vi "01 Reading a voltage.vi"() -> ()   [LabVIEW 2019]
uses:
  <vilib>/Instr/_visa.llb/VISA Configure Serial Port (Instr).vi
panel:
  out "Connected":bool
  in  "stop":bool
  in  "Arduino code":string="/*\n  Analog input, analog output, serial output\n\n  Reads an analog input pin, maps the result to a range from 0 to 255 and uses\n  the result to set the pulse width modulation (PWM) of an output pin.\n  Also prints the results to the Serial Monitor.\n\n  The circuit:\n  - potentiometer connected to analog pin 0.\n    Center pin of the potentiometer goes to the analog pin.\n    side pins of the potentiometer go to +5V and ground\n  - LED connected from digital pin 9 to ground\n\n  created 29 Dec. 2008\n  modified 9 Apr 2012\n  by Tom Igoe\n\n  This example code is in the public domain.\n\n  http://www.arduino.cc/en/Tutorial/AnalogInOutSerial\n*/\n\n// These constants won't change. They're used to give names to the pins used:\nconst int analogInPin = A0;  // Analog input pin that the potentiometer is attached to\nconst int analogOutPin = 9; // Analog output pin that the LED is attached to\n\nint sensorValue = 0;        // value read from the pot\nint outputValue = 0;        // value output to the PWM (analog out)\n\nvoid setup() {\n  // initialize serial communications at 9600 bps:\n  Serial.begin(9600);\n}\n\nvoid loop() {\n  // read the analog in value:\n  sensorValue = analogRead(analogInPin);\n  // map it to the range of the analog out:\n  outputValue = map(sensorValue, 0, 1023, 0, 255);\n  // change the analog out value:\n  analogWrite(analogOutPin, outputValue);\n\n  // print the results to the Serial Monitor:\n  Serial.print(\"sensor = \");\n  Serial.print(sensorValue);\n  Serial.print(\"\\t output = \");\n  Serial.println(outputValue);\n\n  // wait 2 milliseconds before the next loop for the analog-to-digital\n  // converter to settle after the last reading:\n  delay(2);\n}"
  in  "Arduino Port":refnum<visa-resource-name>
  out "Gauge":i32(knob) scale=0.0..1000.0
  # "Download and run the Arduino Example Code AnalogInOutSerial (below)\nHit the Run arrow and see the Gauge change to the value of the sensor (read over serial)"
  # "Hit Cmd E to see the diagram (code)"
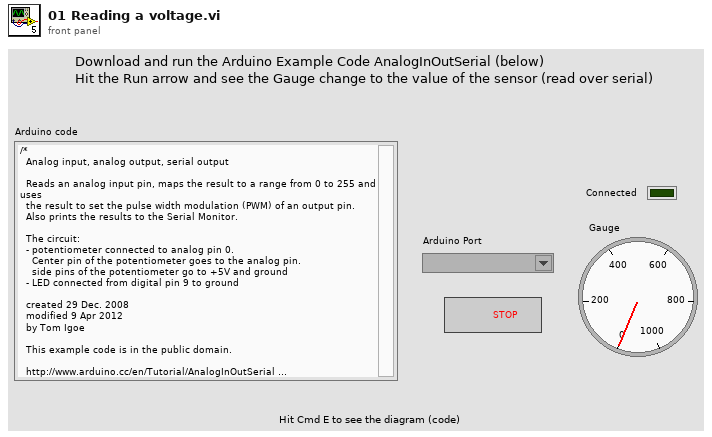
[diagram p1: front panel]
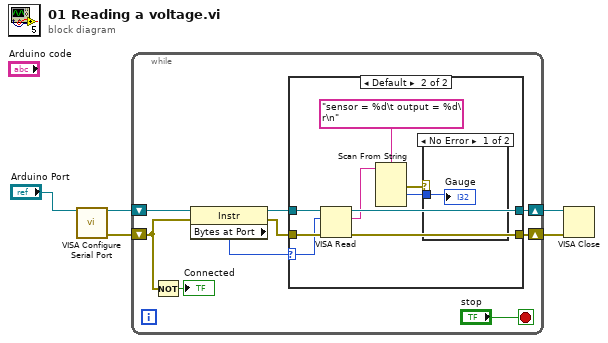
[diagram p0: block diagram]
diagram:
  n1 = call-poly "VISA Configure Serial Port"("VISA resource name"="Arduino Port") -> ("VISA resource name out"=w4:refnum<visa-resource-name>, "error out"=w3:errorcluster)  [unwired: 13 in]
  n2 = while {
    shift-right: [w10] -> w1
    shift-left: w4 -> [w14]
    shift-right: [w11] -> w2
    shift-left: w3 -> [w7]
    stop <- "stop" stop-if-true
    n3 = Not(x=w7) -> (.not. x?=→"Connected":bool)
    n4 = property class="Instr"(reference=w14, error in=w7) -> (reference out=w13:refnum<visa-resource-name>, error out=w12:errorcluster, "Bytes at Port"=w8:u32)
    n5 = case shown="Default" w8 {
      selector: w8 -> [_ w21]
      tunnel: w13 -> [w16 w25]
      tunnel: w12 -> [w15 w24]
      tunnel: [w15 w23] -> w11
      tunnel: [w16 w22] -> w10
      frame 0 {
      }
      frame Default {
        n6 = VISA Read(VISA resource name=w25, byte count=w21, error in (no error)=w24) -> (VISA resource name out=w22:refnum<visa-resource-name>, read buffer=w19:string, error out=w23:errorcluster)  [unwired: 1 out]
        n7 = Scan From String(format string="sensor = %d\t output = %d\r\n", input string=w19) -> (error out=w18:errorcluster, output 1=w17:i32)  [unwired: 5 in, 2 out]
        n8 = case shown="No Error" w18 {
          tunnel: w17 -> [w26 _]
          frame No Error {
            "Gauge" <- w26
          }
          frame Error {
          }
        }
      }
    }
  }
  n9 = VISA Close(VISA resource name=w1, error in (no error)=w2) -> ()  [unwired: 1 out]
